vi "Conf DIO Alarm.vi"(0 "VISA Resource Name":refnum<visa-resource-name>, 1 "Enable Alarm? (T: Enable)":bool=TRUE, 2 "Set/Check (F: Set)":bool, 3 "Polarity (T: Positive)":bool=TRUE, 4 "Mode (F: Track)":bool, 5 "error in (no error)":errorcluster, 6 "Comparison Mode (T: Equal)":bool=TRUE, 7 "Pattern (0)":u16, 8 "Channel List(empty)":string, 9 "Mask (0)":u16, 10 "Bits (F: 8) - Deprecated":bool, 11 "Clear Bit (5:None)":enum16{"1", "2", "3", "4", "All", "None"}(ring)=enum."None", 12 "Check (0:Alarm #)":u16(ring) items=["Alarm #"=0, "Polarity"=1, "State"=2, "Comparison Mode"=3, "Pattern (8 Bit)"=4, "Mask (8 Bit)"=5, "Alarm Mode"=8], 13 "Output # (1)":enum16{"1", "2", "3", "4"}(ring)) -> (14 "VISA Resource Name Out":refnum<visa-resource-name>, 16 "Configuration?":string, 19 "error out":errorcluster)   [LabVIEW 2016, in "Agilent 34970.lvlib"]
doc: "This VI lets you configure or check alarms on the specified DIO channels."
uses:
  Agilent 34970.lvlib
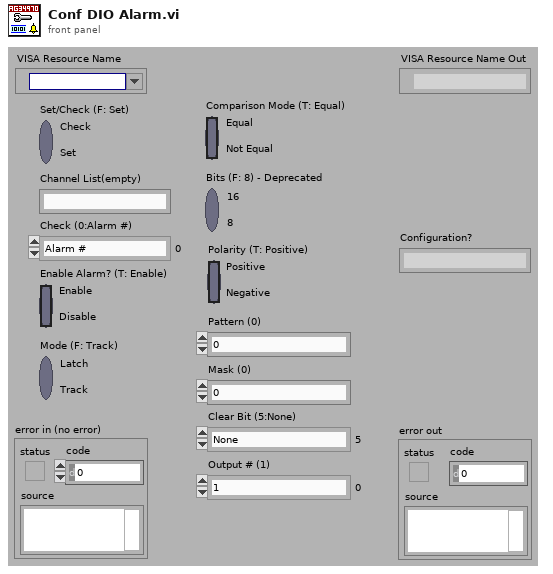
[diagram p1: front panel]
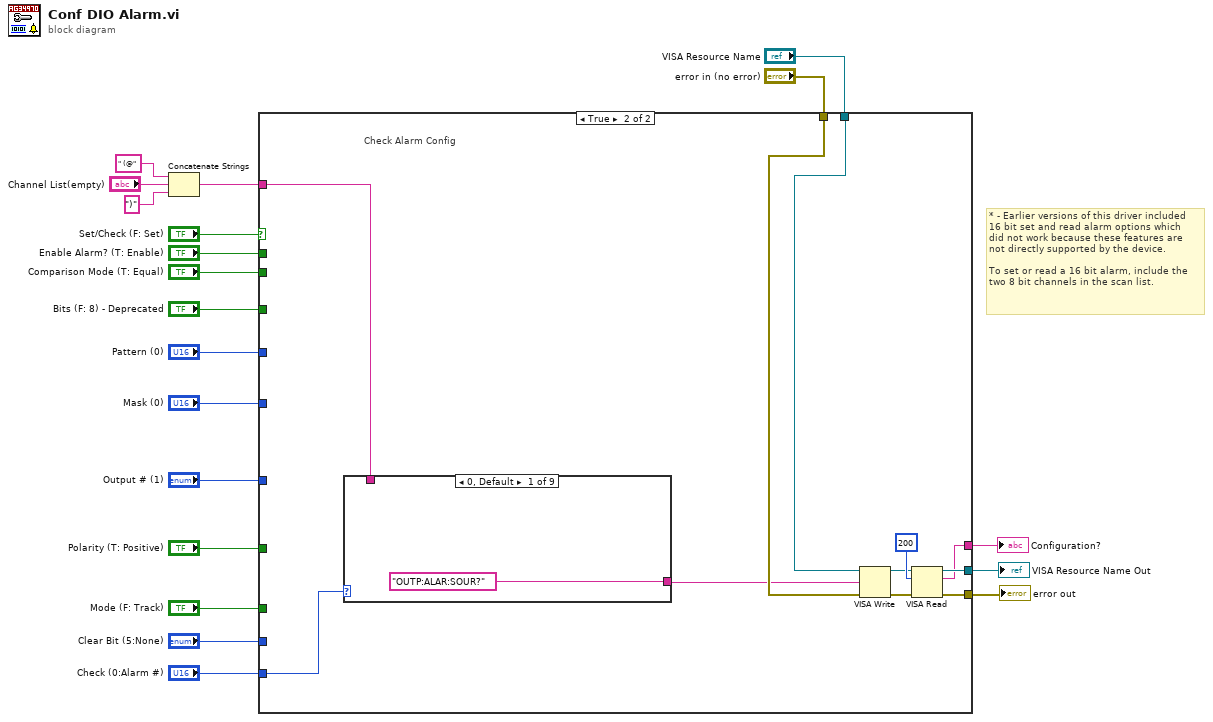
[diagram p0: block diagram]
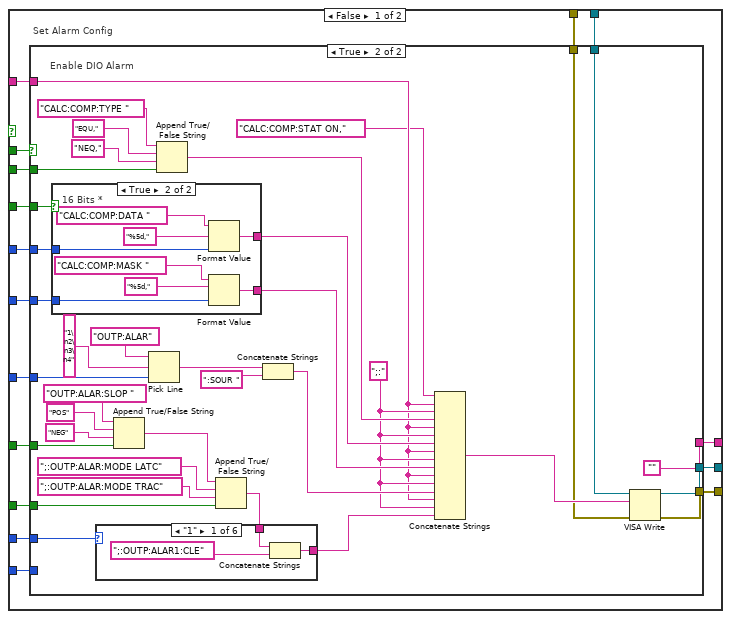
[diagram p2: hidden frame]
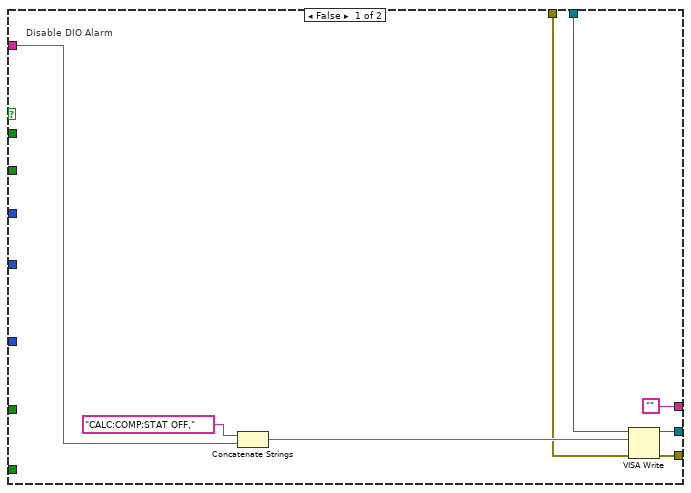
[diagram p3: hidden frame]
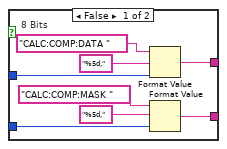
[diagram p4: hidden frame]
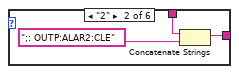
[diagram p5: hidden frame]
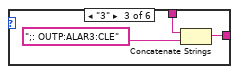
[diagram p6: hidden frame]
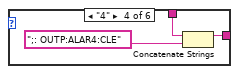
[diagram p7: hidden frame]
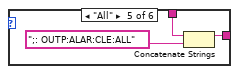
[diagram p8: hidden frame]
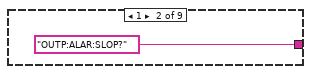
[diagram p10: hidden frame]
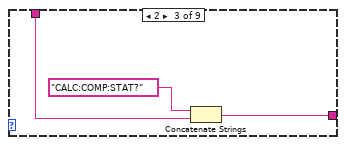
[diagram p11: hidden frame]
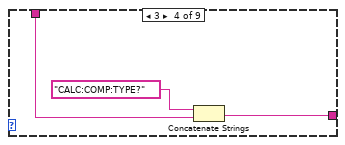
[diagram p12: hidden frame]
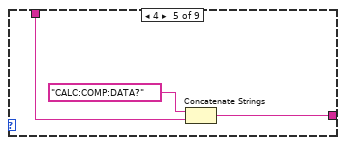
[diagram p13: hidden frame]
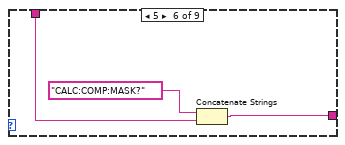
[diagram p14: hidden frame]
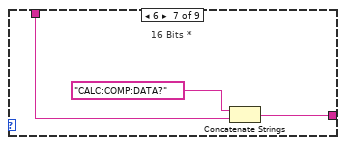
[diagram p15: hidden frame]
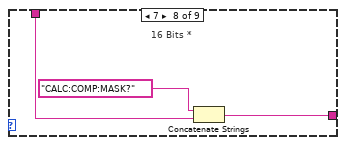
[diagram p16: hidden frame]
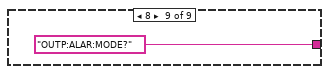
[diagram p17: hidden frame]
diagram:
  # "* - Earlier versions of this driver included\n16 bit set and read alarm options which \ndid not work because these features are \nnot directly supported by the device.  \n\nTo set or read a 16 bit alarm, include the \ntwo 8 bit channels in the scan list."
  n1 = Concatenate Strings(" (@", "Channel List(empty)", ")") -> (w18:string)
  n2 = case shown="True" "Set/Check (F: Set)" {
    tunnel: w18 -> [w36 w120]
    tunnel: [w35 w119] -> w5
    tunnel: [w34 w118] -> w4
    tunnel: [w33 w117] -> w17
    tunnel: "Enable Alarm? (T: Enable)" -> [w32 _]
    tunnel: "Output # (1)" -> [w31 _]
    tunnel: "Polarity (T: Positive)" -> [w30 _]
    tunnel: "Mode (F: Track)" -> [w29 _]
    tunnel: "Clear Bit (5:None)" -> [w28 _]
    tunnel: "Check (0:Alarm #)" -> [w27 w116]
    tunnel: "Comparison Mode (T: Equal)" -> [w26 _]
    tunnel: "Bits (F: 8) - Deprecated" -> [w25 _]
    tunnel: "Pattern (0)" -> [w24 _]
    tunnel: "Mask (0)" -> [w23 _]
    tunnel: "VISA Resource Name" -> [w22 w114]
    tunnel: "error in (no error)" -> [w21 w115]
    frame False {
      # "Set Alarm Config"
      n3 = case shown="True" w32 {
        tunnel: w36 -> [w42 w50]
        tunnel: [w41 w80] -> w35
        tunnel: [w39 w79] -> w34
        tunnel: ["" ""] -> w33
        tunnel: w31 -> [_ w75]
        tunnel: w30 -> [_ w71]
        tunnel: w29 -> [_ w69]
        tunnel: w28 -> [_ w68]
        tunnel: w27 -> [_ _]
        tunnel: w26 -> [_ w58]
        tunnel: w25 -> [_ w57]
        tunnel: w24 -> [_ w56]
        tunnel: w23 -> [_ w55]
        tunnel: w22 -> [w37 w47]
        tunnel: w21 -> [w38 w46]
        frame False {
          # "Disable DIO Alarm"
          n4 = Concatenate Strings("CALC:COMP:STAT OFF,", w42) -> (w43:string)
          n5 = VISA Write(VISA resource name=w37, write buffer=w43, error in (no error)=w38) -> (VISA resource name out=w41:refnum<visa-resource-name>, error out=w39:errorcluster)  [unwired: 1 out]
        }
        frame True {
          w51 = ";:"
          # "Enable DIO Alarm"
          n6 = case shown="True" w57 {
            tunnel: w56 -> [w88 w93]
            tunnel: w55 -> [w87 w92]
            tunnel: [w82 w89] -> w54
            tunnel: [w81 w90] -> w53
            frame False {
              # "8 Bits"
              n7 = Format Value(string ("")="CALC:COMP:DATA ", format string="%5d,", value (0)=w88) -> (output string=w81:string)
              n8 = Format Value(string ("")="CALC:COMP:MASK ", format string="%5d,", value (0)=w87) -> (output string=w82:string)
            }
            frame True {
              # "16 Bits *"
              n9 = Format Value(string ("")="CALC:COMP:DATA ", format string="%5d,", value (0)=w93) -> (output string=w90:string)
              n10 = Format Value(string ("")="CALC:COMP:MASK ", format string="%5d,", value (0)=w92) -> (output string=w89:string)
            }
          }
          n11 = Append True/False String(1:w71, 2:"NEG", 3:"POS", 4:"OUTP:ALAR:SLOP ") -> (0:w70:string)
          n12 = Pick Line(string ("")="OUTP:ALAR", multi-line string="1\n2\n3\n4", line index=w75) -> (output string=w74:string)
          n13 = Append True/False String(1:w58, 2:"NEQ,", 3:"EQU,", 4:"CALC:COMP:TYPE ") -> (0:w52:string)
          n14 = Append True/False String(1:w69, 2:";:OUTP:ALAR:MODE TRAC", 3:";:OUTP:ALAR:MODE LATC", 4:w70) -> (0:w67:string)
          n15 = case shown="\"1\"" w68 {
            tunnel: w67 -> [w99 w101 w104 w107 w110 w112]
            tunnel: [w97 w100 w103 w106 w109 w112] -> w66
            frame "1" {
              n16 = Concatenate Strings(w99, ";:OUTP:ALAR1:CLE") -> (w97:string)
            }
            frame "2" {
              n17 = Concatenate Strings(w101, ";: OUTP:ALAR2:CLE") -> (w100:string)
            }
            frame "3" {
              n18 = Concatenate Strings(w104, ";: OUTP:ALAR3:CLE") -> (w103:string)
            }
            frame "4" {
              n19 = Concatenate Strings(w107, ";: OUTP:ALAR4:CLE") -> (w106:string)
            }
            frame "All" {
              n20 = Concatenate Strings(w110, ";: OUTP:ALAR:CLE:ALL") -> (w109:string)
            }
            frame "None" {
            }
          }
          n21 = Concatenate Strings(w74, ":SOUR ") -> (w65:string)
          n22 = Concatenate Strings("CALC:COMP:STAT ON,", w50, w51, w52, w50, w51, w53, w50, w51, w54, w50, w51, w65, w50, w51, w66) -> (w48:string)
          n23 = VISA Write(VISA resource name=w47, write buffer=w48, error in (no error)=w46) -> (VISA resource name out=w80:refnum<visa-resource-name>, error out=w79:errorcluster)  [unwired: 1 out]
        }
      }
    }
    frame True {
      # "Check Alarm Config"
      n24 = case shown="0, Default" w116 {
        tunnel: w120 -> [_ _ w127 w129 w133 w135 w139 w143 _]
        tunnel: ["OUTP:ALAR:SOUR?" "OUTP:ALAR:SLOP?" w126 w130 w132 w136 w138 w142 "OUTP:ALAR:MODE?"] -> w113
        frame 0, Default {
        }
        frame 1 {
        }
        frame 2 {
          n25 = Concatenate Strings("CALC:COMP:STAT?", w127) -> (w126:string)
        }
        frame 3 {
          n26 = Concatenate Strings("CALC:COMP:TYPE?", w129) -> (w130:string)
        }
        frame 4 {
          n27 = Concatenate Strings("CALC:COMP:DATA?", w133) -> (w132:string)
        }
        frame 5 {
          n28 = Concatenate Strings("CALC:COMP:MASK?", w135) -> (w136:string)
        }
        frame 6 {
          # "16 Bits *"
          n29 = Concatenate Strings("CALC:COMP:DATA?", w139) -> (w138:string)
        }
        frame 7 {
          # "16 Bits *"
          n30 = Concatenate Strings("CALC:COMP:MASK?", w143) -> (w142:string)
        }
        frame 8 {
        }
      }
      n31 = VISA Write(VISA resource name=w114, write buffer=w113, error in (no error)=w115) -> (VISA resource name out=w122:refnum<visa-resource-name>, error out=w121:errorcluster)  [unwired: 1 out]
      n32 = VISA Read(VISA resource name=w122, byte count=u32 200 ("byte count (0)"), error in (no error)=w121) -> (VISA resource name out=w119:refnum<visa-resource-name>, read buffer=w117:string, error out=w118:errorcluster)  [unwired: 1 out]
    }
  }
  "Configuration?" <- w17
  "VISA Resource Name Out" <- w5
  "error out" <- w4
